vi "fit aois.vi"(5 "End frame":u32, 6 "White level":dbl format="%.2f", 7 "Header Info":T2 {"Pixel depth" items=["8 bits", "16 bits", "Float", "Complex", "RGB", "HSL"]; "time of 1st frame, \nsec since 1/1/04" format="%.2f"}, 8 "Start frame":u32, 9 "Black level":dbl format="%.2f", 10 "Acquisition refnum array":refnum<file>[](array[refnum])) -> ()   [LabVIEW 2016]
doc: "Tracks objects in successive frames of a video by calculating the parameter values that give the best fit between an analytical function and the portions of the image in selected areas of interest.\n\nOutputs an HTML report summarizing the fitting run, and a CSV-format file (which can be read by spreadsheet programs) containing the results. In addition to the parameters, each row the CSV file also contains:\n\nframe -- frame number\naoi -- aoi number\ntime -- time in milliseconds\nmse -- mean square error of the fit (or -1 if it didn't fit)\nintegral -- sum of the pixels in the aoi"
uses:
  Header file data.ctl
  Seq file v 1/Offset table.ctl
  Seq file v 1/Offset.ctl
  Seq file v 1/file number.ctl
  Parameter array.ctt
  Fit type setup.ctt
  <vilib>/Utility/NIReport.llb/HTML Report Text Alignment.ctl
  <vilib>/Utility/NIReport.llb/HTML Report Image Alignment.ctl
  AOI List Globals.vi
  GLIMPSE Globals.vi
  <vilib>/Utility/NIReport.llb/Append Report Text (str wrap).vi
  <vilib>/Utility/NIReport.llb/Append Image to Report (string wrap).vi
  <vilib>/Utility/NIReport.llb/NI_report.lvclass
  <vilib>/vision/NI_Vision_Development_Module.lvlib
  <vilib>/Utility/NIReport.llb/NI_ReportGenerationCore.lvlib
panel:
  in  "Write record when no fit?":bool=TRUE
  out "Fit":dbl[](array[numeric])
  in  "max iterations":i32=200
  in  "Update graphics?":bool=TRUE
  in  "Fit type":u16(ring) items=["2D Gaussian", "AOI Stats Only", "2D Gaussian 2 width", "Difference of Offset Gaussians (DIC)"]
  in  "Move AOIs?":bool=TRUE
  out "Last error":string
  in  "Parameters":T1=[{"Name"="bk", "Specify IV?"=TRUE, "Initial Val."=-30000.0, "Lower lim."=-32768.0, "Upper lim."=32767.0, "Fit?"=TRUE}, {"Name"="ht", "Specify IV?"=TRUE, "Initial Val."=1000.0, "Lower lim."=1.0, "Upper lim."=65000.0, "Fit?"=TRUE}, {"Name"="xc", "Specify IV?"=TRUE, "Initial Val."=10.0, "Lower lim."=0.0, "Upper lim."=512.0, "Fit?"=TRUE}, {"Name"="yc", "Specify IV?"=TRUE, "Initial Val."=10.0, "Lower lim."=0.0, "Upper lim."=512.0, "Fit?"=TRUE}, {"Name"="wi", "Specify IV?"=TRUE, "Initial Val."=2.0, "Lower lim."=0.5, "Upper lim."=20.0, "Fit?"=TRUE}] {"Upper lim." format="%.2f"; "Lower lim." format="%.2f"; "Initial Val." format="%.2f"}
  out "MSEs":dbl[](graph)
  in  "Go":bool
  out "AOI Number":i32(slide) scale=1.0..2.0
  out "Frame Number":i32(slide) scale=1.0..4390.0
  in  "stop":bool
  # "These parameters not for interactive use"
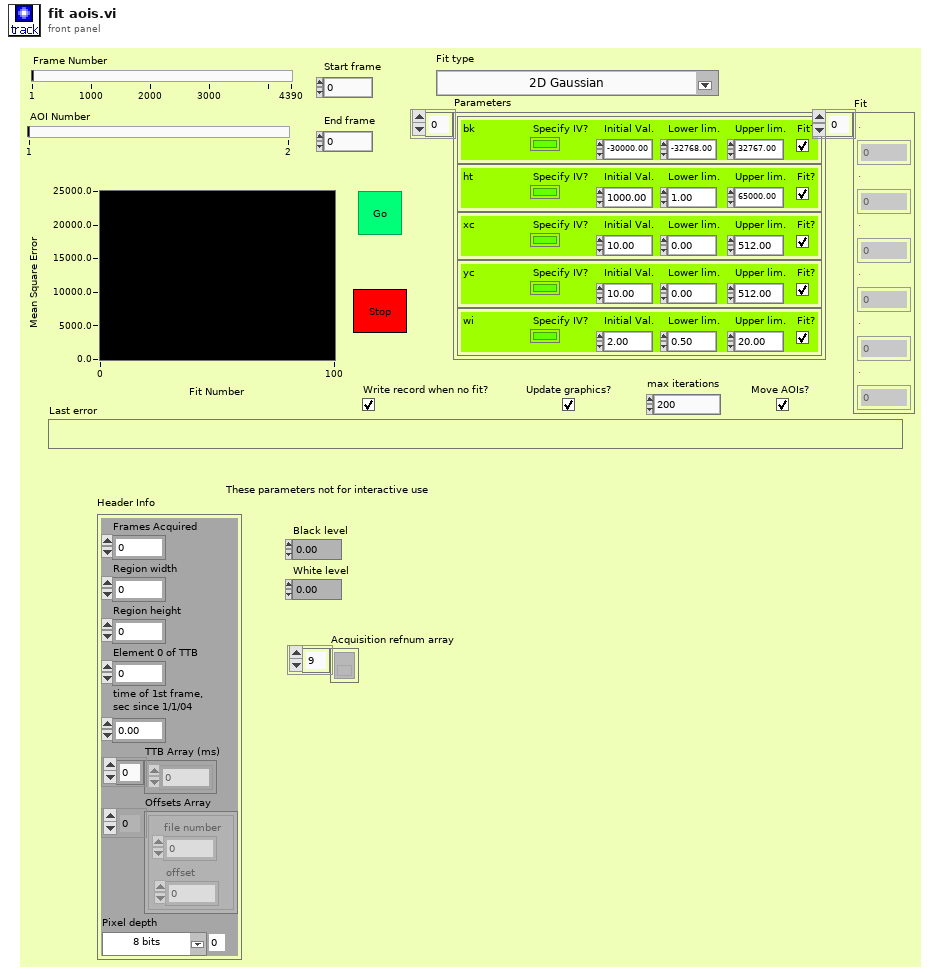
[diagram p1: front panel]
types:
  T1 = typedef "Parameter array.ctt" = cluster{"Name":string, "Specify IV?":bool, "Initial Val.":dbl, "Lower lim.":dbl, "Upper lim.":dbl, "Fit?":bool}[]
  T2 = typedef "Header file data.ctl" = cluster{"Frames Acquired":u32, "Region width":i32, "Region height":i32, "Element 0 of TTB":u32, "time of 1st frame, \nsec since 1/1/04":dbl, "TTB Array (ms)":u32[], "Offsets Array":T3, "Pixel depth":u32}
  T3 = typedef "Offset table.ctl" = cluster{"offset":T4, "file number":T5}[]
  T4 = typedef "Offset.ctl" = i32
  T5 = typedef "file number.ctl" = u8
  T6 = cluster{"Name":string, "Initial val.":dbl, "Fit?":bool}[][]
  T7 = typedef "Fit type setup.ctt" = cluster{"Fit type":string, "derivative":u16, "Parameters":T1}
  T8 = enum16{"open", "open or create", "create or replace", "create", "open (read only)"}
  T9 = typedef "IMAQ Image.ctl" = refnum<image>
  T10 = typedef "Generate Report Object Reference.ctl" = refnum<class "NI_report.lvclass">
  T11 = typedef "NI_ReportGenerationCore.lvlib/HTML Report Image Alignment.ctl" = enum16{"(default)", "LEFT", "RIGHT", "TOP", "TEXTTOP", "MIDDLE", "ABSMIDDLE", "BASELINE", "BOTTOM", "ABSBOTTOM"}
  T12 = typedef "NI_ReportGenerationCore.lvlib/HTML Report Text Alignment.ctl" = enum16{"(default)", "LEFT", "CENTER", "RIGHT"}
  T13 = cluster{"Name":string, "Initial val.":dbl, "Fit?":bool}[]
  T14 = cluster{"Name":string, "Initial Val.":dbl, "Fit?":bool}
  T15 = cluster{"Name":string, "Value":dbl, "Fit?":bool}[]
  T16 = cluster{"Name":string, "Initial Val.":dbl, "Fit?":bool}[]
  T17 = cluster{"AOI List[0]":u16, "AOI List[1]":u16, "AOI List[2]":u16, "AOI List[3]":u16, "AOI List[4]":u16, "AOI List[5]":u16, "AOI List[6]":u16, "AOI List[7]":u16, "AOI List[8]":u16}
  T18 = cluster{"AOI List[0]":u16, "AOI List[1]":u16, "AOI List[2]":u16, "AOI List[3]":u16}
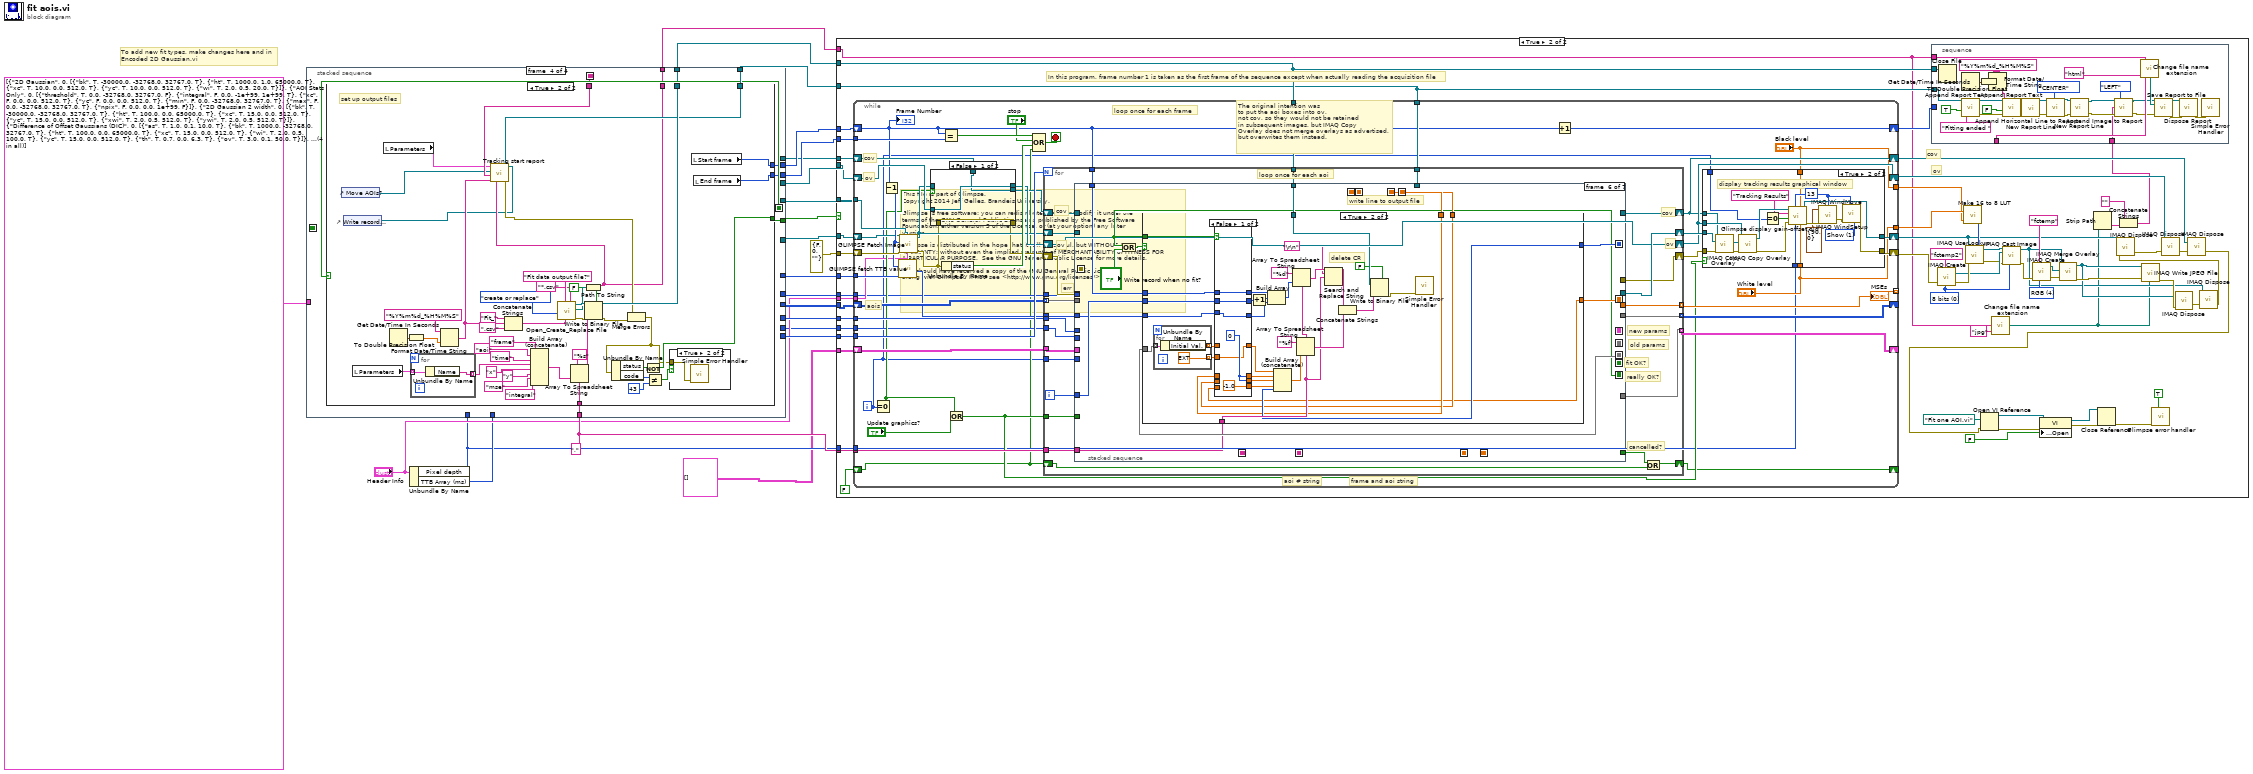
[diagram p0: block diagram]
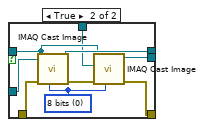
[diagram p4: hidden frame]
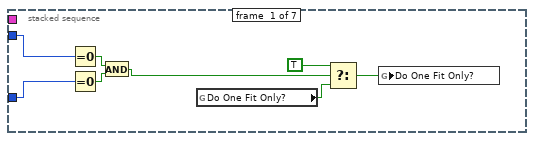
[diagram p5: hidden frame]
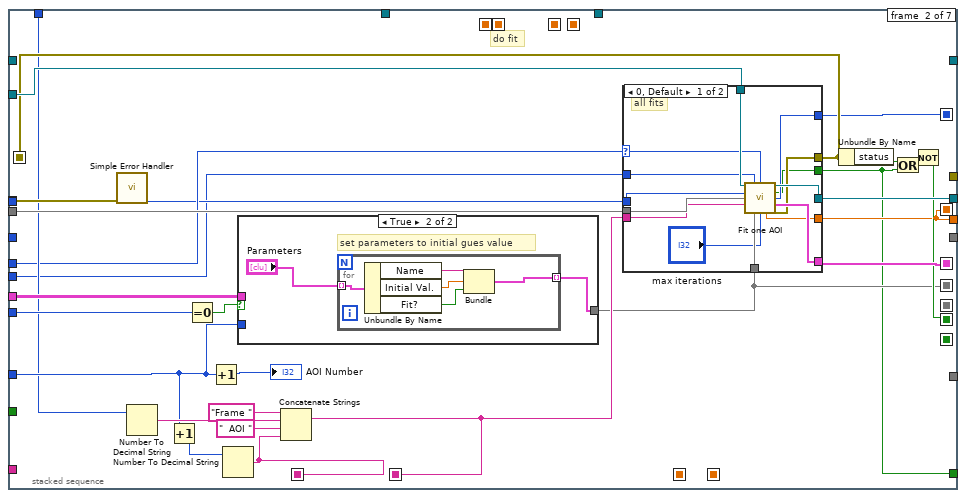
[diagram p6: hidden frame]
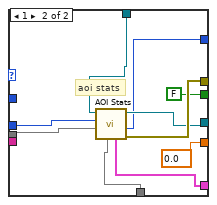
[diagram p7: hidden frame]
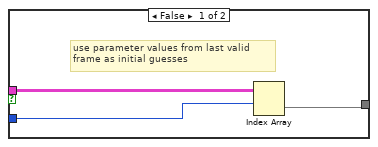
[diagram p8: hidden frame]
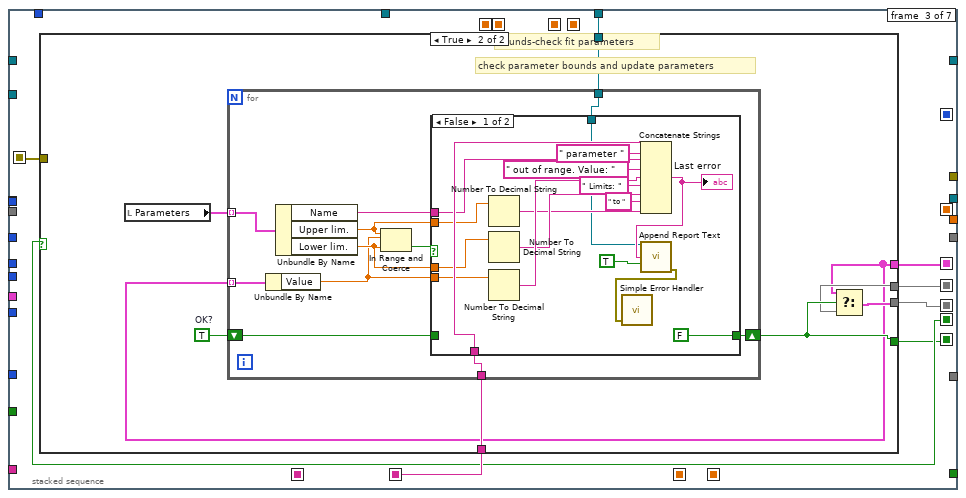
[diagram p9: hidden frame]
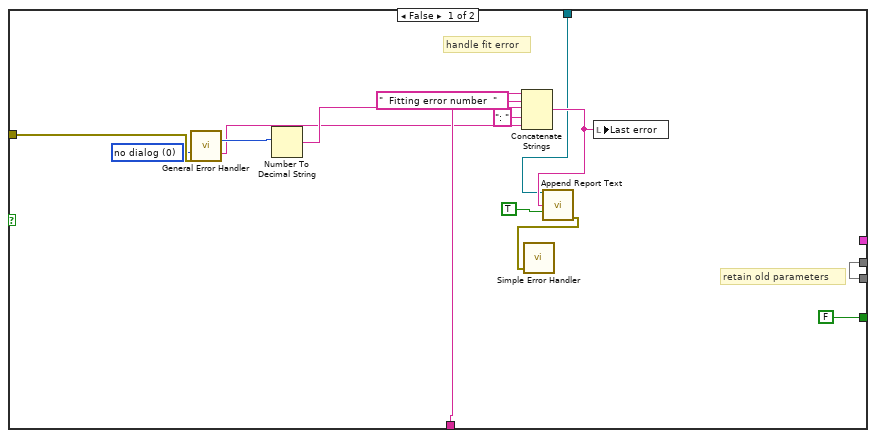
[diagram p10: hidden frame]
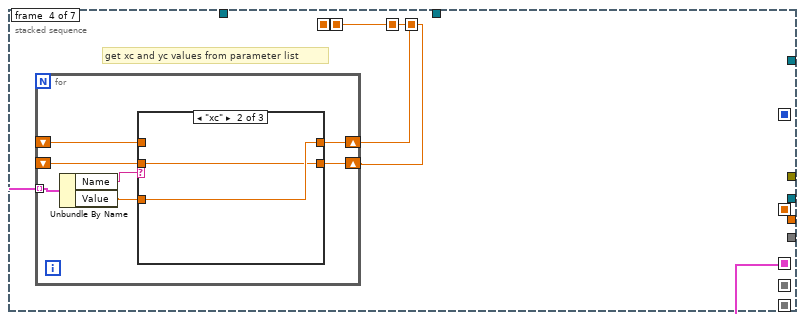
[diagram p12: hidden frame]
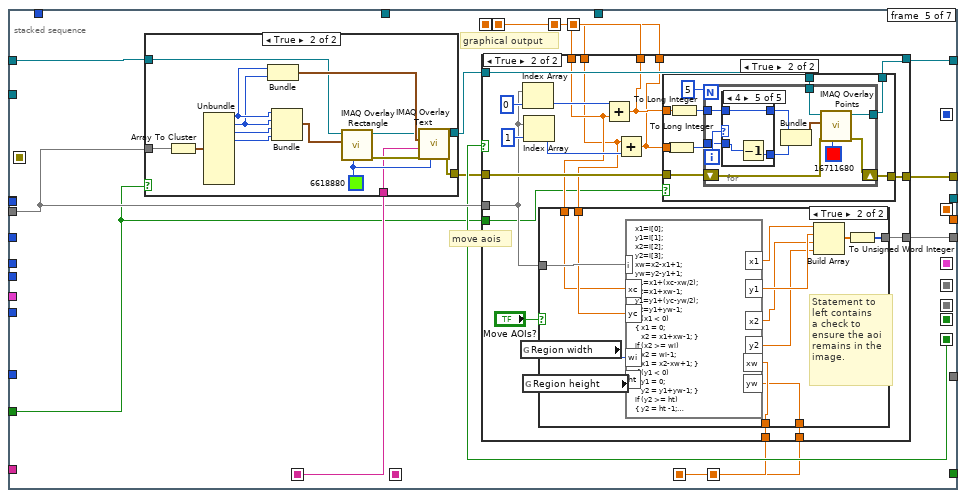
[diagram p15: hidden frame]
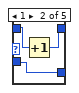
[diagram p20: hidden frame]
diagram:
  w9 = "," ("delimiter (Tab)")
  # "This file is part of Glimpse. \nCopyright 2014 Jeff Gelles, Brandeis University.    \n\nGlimpse is free software: you can redistribute it and/or modify it under the \nterms of the GNU General Public License as published by the Free Software \nFoundation, either version 3 of the License, or (at your option) any later \nversion.\n\nGlimpse is distributed in the hope that it will be useful, but WITHOUT ANY \nWARRANTY; without even the implied warranty of MERCHANTABILITY or FITNESS FOR \nA PARTICULAR PURPOSE.  See the GNU General Public License for more details.\n\nYou should have received a copy of the GNU General Public License\nalong with Glimpse.  If not, see <http://www.gnu.org/licenses/>."
  # "To add new fit types, make changes here and in\nEncoded 2D Gaussian.vi"
  n1 = Unbundle By Name("Header Info") -> ("Pixel depth"=w3:u32, "TTB Array (ms)"=w5:u32[])
  n2 = stacked-sequence {
    seq-local: [_ w43 _ _] -> [_ _ w60 _]
    seq-local: [_ _ w59 _] -> [_ _ _ w83]
    seq-local: [_ _ w55 _] -> [_ _ _ w78]
    tunnel: [_ _ _ w76] -> w23
    tunnel: [_ "Acquisition refnum array" _ _] -> w22
    tunnel: [_ w50 _ _] -> w21
    tunnel: [_ w32 _ _] -> w20
    tunnel: [_ _ _ w77] -> w19
    tunnel: [_ w47 _ _] -> w18
    tunnel: [_ _ _ w82] -> w17
    tunnel: [_ w40 _ _] -> w16
    tunnel: [_ w36 _ _] -> w14
    tunnel: [_ w33 _ _] -> w13
    tunnel: [_ _ _ w84] -> w12
    tunnel: [_ _ _ w81] -> w11
    tunnel: [_ _ _ w80] -> w10
    tunnel: w9 -> [_ _ _ w79]
    tunnel: T7[] [{"Fit type"="2D Gaussian", "derivative"=0, "Parameters"=[{"Name"="bk", "Specify IV?"=TRUE, "Initial Val."=-30000.0, "Lower lim."=-32768.0, "Upper lim."=32767.0, "Fit?"=TRUE}, {"Name"="ht", "Specify IV?"=TRUE, "Initial Val."=1000.0, "Lower lim."=1.0, "Upper lim."=65000.0, "Fit?"=TRUE}, {"Name"="xc", "Specify IV?"=TRUE, "Initial Val."=10.0, "Lower lim."=0.0, "Upper lim."=512.0, "Fit?"=TRUE}, {"Name"="yc", "Specify IV?"=TRUE, "Initial Val."=10.0, "Lower lim."=0.0, "Upper lim."=512.0, "Fit?"=TRUE}, {"Name"="wi", "Specify IV?"=TRUE, "Initial Val."=2.0, "Lower lim."=0.5, "Upper lim."=20.0, "Fit?"=TRUE}]}, {"Fit type"="AOI Stats Only", "derivative"=0, "Parameters"=[{"Name"="threshold", "Specify IV?"=TRUE, "Initial Val."=0.0, "Lower lim."=-32768.0, "Upper lim."=32767.0, "Fit?"=FALSE}, {"Name"="integral", "Specify IV?"=FALSE, "Initial Val."=0.0, "Lower lim."=-1e+99, "Upper lim."=1e+99, "Fit?"=TRUE}, {"Name"="xc", "Specify IV?"=FALSE, "Initial Val."=0.0, "Lower lim."=0.0, "Upper lim."=512.0, "Fit?"=TRUE}, {"Name"="yc", "Specify IV?"=FALSE, "Initial Val."=0.0, "Lower lim."=0.0, "Upper lim."=512.0, "Fit?"=TRUE}, {"Name"="min", "Specify IV?"=FALSE, "Initial Val."=0.0, "Lower lim."=-32768.0, "Upper lim."=32767.0, "Fit?"=TRUE}, {"Name"="max", "Specify IV?"=FALSE, "Initial Val."=0.0, "Lower lim."=-32768.0, "Upper lim."=32767.0, "Fit?"=TRUE}, {"Name"="npix", "Specify IV?"=FALSE, "Initial Val."=0.0, "Lower lim."=0.0, "Upper lim."=1e+99, "Fit?"=FALSE}]}, {"Fit type"="2D Gaussian 2 width", "derivative"=0, "Parameters"=[{"Name"="bk", "Specify IV?"=TRUE, "Initial Val."=-30000.0, "Lower lim."=-32768.0, "Upper lim."=32767.0, "Fit?"=TRUE}, {"Name"="ht", "Specify IV?"=TRUE, "Initial Val."=100.0, "Lower lim."=0.0, "Upper lim."=65000.0, "Fit?"=TRUE}, {"Name"="xc", "Specify IV?"=TRUE, "Initial Val."=15.0, "Lower lim."=0.0, "Upper lim."=512.0, "Fit?"=TRUE}, {"Name"="yc", "Specify IV?"=TRUE, "Initial Val."=15.0, "Lower lim."=0.0, "Upper lim."=512.0, "Fit?"=TRUE}, {"Name"="xwi", "Specify IV?"=TRUE, "Initial Val."=2.0, "Lower lim."=0.5, "Upper lim."=512.0, "Fit?"=TRUE}, {"Name"="ywi", "Specify IV?"=TRUE, "Initial Val."=2.0, "Lower lim."=0.5, "Upper lim."=512.0, "Fit?"=TRUE}]}, {"Fit type"="Difference of Offset Gaussians (DIC)", "derivative"=0, "Parameters"=[{"Name"="as", "Specify IV?"=TRUE, "Initial Val."=1.0, "Lower lim."=0.1, "Upper lim."=10.0, "Fit?"=TRUE}, {"Name"="bk", "Specify IV?"=TRUE, "Initial Val."=1000.0, "Lower lim."=-32768.0, "Upper lim."=32767.0, "Fit?"=TRUE}, {"Name"="ht", "Specify IV?"=TRUE, "Initial Val."=100.0, "Lower lim."=0.0, "Upper lim."=65000.0, "Fit?"=TRUE}, {"Name"="xc", "Specify IV?"=TRUE, "Initial Val."=15.0, "Lower lim."=0.0, "Upper lim."=512.0, "Fit?"=TRUE}, {"Name"="wi", "Specify IV?"=TRUE, "Initial Val."=2.0, "Lower lim."=0.5, "Upper lim."=100.0, "Fit?"=TRUE}, {"Name"="yc", "Specify IV?"=TRUE, "Initial Val."=15.0, "Lower lim."=0.0, "Upper lim."=512.0, "Fit?"=TRUE}, {"Name"="th", "Specify IV?"=TRUE, "Initial Val."=0.7, "Lower lim."=0.0, "Upper lim."=6.3, "Fit?"=TRUE}, {"Name"="ov", "Specify IV?"=TRUE, "Initial Val."=3.0, "Lower lim."=0.1, "Upper lim."=50.0, "Fit?"=TRUE}]}] -> [w25 _ w57 _]
    tunnel: [_ _ w56 _] -> w7
    tunnel: w3 -> [_ w31 _ _]
    tunnel: w5 -> [_ w32 _ _]
    tunnel: [_ w31 _ _] -> w4
    tunnel: [_ _ w53 _] -> w1
    frame #0 {
      n3 = for {
        tunnel: w25 -> [w29] mode=indexing
        tunnel: [w28] -> w24 mode=indexing
        n4 = Unbundle By Name(w29) -> ("Fit type"=w28:string)
      }
      n5 = property on="Fit type" class="Ring (strict)"("Strings []"=w24) -> ()  [unwired: 2 in, 2 out]
      n6 = local write "stop"(FALSE ("stop")) -> ()
      n7 = local write "Go"(FALSE ("stop")) -> ()
    }
    frame #1 {
      w34 = u32 0 items=["8 bits", "16 bits", "Float", "Complex", "RGB", "HSL"] ("Image Type")
      n8 = global read "AOI List Globals.vi" "AOI List"() -> (w47:u16[][])
      n9 = property on="Frame Number" class="Slide (strict)"("Scale.Range:Minimum"="Start frame", "Scale.Range:Maximum"="End frame") -> ()  [unwired: 2 in, 2 out]
      n10 = call "Position calling vi to LR 2.vi"("Corner"=enum16{"LR", "LL"}."LL") -> ()  [unwired: 1 in, 4 out]
      n11 = call "IMAQ Create"("Image Name"="cum overlay", "Image Type"=w34) -> ("New Image"=w33:T9)  [unwired: 2 in, 2 out]
      n12 = Array Size(array=w47) -> (size(s)=w46:i32[])
      n13 = Index Array(array=w46, index=0) -> (element=w40:i32)
      n14 = local write "Frame Number"(0 ("Frame Number")) -> ()
      n15 = local write "AOI Number"(0 ("AOI Number")) -> ()
      n16 = call "IMAQ Create"("Image Name"="overlay", "Image Type"=w34) -> ("New Image"=w36:T9, "error out"=w37:errorcluster)  [unwired: 2 in, 1 out]
      n17 = property on="AOI Number" class="Slide (strict)"("Scale.Range:Maximum"=w40, "Scale.Range:Minimum"=1.0) -> ()  [unwired: 2 in, 2 out]
      n18 = call "IMAQ Create"("Image Name"="fitimage", "Image Type"=w31, "error in (no error)"=w37) -> ("New Image"=w50:T9, "error out"=w44:errorcluster)  [unwired: 1 in, 1 out]
      n19 = Unbundle By Name(w44) -> ("status"=w43:bool)
      n20 = call <vilib>:"Simple Error Handler.vi"("error in (no error)"=w44) -> ()  [unwired: 1 in, 8 out]
    }
    frame #2 {
      n21 = local read "Fit type"() -> (w54:u16)
      n22 = while {
        tunnel: w60 -> [w70]
        tunnel: ["Go"] -> w59
        shift-right: [w61] -> w56
        shift-left: w54 -> [w65]
        tunnel: w57 -> [w62]
        stop <- w69 stop-if-true
        n23 = To Word Integer(number="Fit type") -> (16bit integer=w61:i16)
        n24 = local read "stop"() -> (w71:bool)
        n25 = Not Equal?(x=w61, y=w65) -> (x != y?=w63:bool)
        n26 = Or(x=w71, y=w70) -> (x .or. y?=w67:bool)
        n27 = Or(x="Go", y=w67) -> (x .or. y?=w69:bool)
        n28 = case shown="True" w63 {
          tunnel: w62 -> [_ w75]
          tunnel: w61 -> [_ w74]
          frame False {
          }
          frame True {
            n29 = Index Array(array=w75, index=w74) -> (element=w73:T7)
            n30 = Unbundle By Name(w73) -> ("Parameters"=w72:T1)
            n31 = local write "Parameters"(w72) -> ()
          }
        }
        n32 = Wait (ms)(milliseconds to wait=u32 300) -> ()  [unwired: 1 out]
      }
      n33 = Index Array(array=w57, index=w56) -> (element=w58:T7)
      n34 = Unbundle By Name(w58) -> ("Fit type"=w55:string, "derivative"=w53:u16)
    }
    frame #3 {
      n35 = case shown="True" w83 {
        selector: w83 -> [w85 _]
        tunnel: [_ w97] -> w84
        tunnel: [w85 w117] -> w82
        tunnel: [_ w104] -> w81
        tunnel: [_ w92] -> w80
        tunnel: w79 -> [_ w102]
        tunnel: w78 -> [_ w95]
        tunnel: [_ w89] -> w77
        tunnel: [_ w88] -> w76
        frame False {
        }
        frame True {
          # "set up output files"
          n36 = control-ref of="Move AOIs?"() -> (w94:refnum<vi>)
          n37 = control-ref of="Write record when no fit?"() -> (w87:refnum<vi>)
          n38 = local read "Parameters"() -> (w116:T1)
          n39 = local read "Parameters"() -> (w93:T1)
          n40 = Get Date/Time In Seconds() -> (seconds since 1Jan1904=w91:timestamp)
          n41 = To Double Precision Float(number=w91) -> (double precision float=w129:dbl)
          n42 = for {
            tunnel: w116 -> [w131] mode=indexing
            tunnel: [w130] -> w110 mode=indexing
            n43 = Unbundle By Name(w131) -> ("Name"=w130:string)
          }
          n44 = Format Date/Time String(time format string (%c)="%Y%m%d_%H%M%S", seconds (now)=w129) -> (date/time string=w124:string)  [unwired: 1 out]
          n45 = Concatenate Strings("Fit_", w124, ".csv" ("string")) -> (w122:string)
          n46 = Build Array (concatenate)("frame", "aoi", "time", w110, "x", "y", "mse", "integral" ("element")) -> (w112:string[])
          n47 = call <vilib>:"Open_Create_Replace File.vi"("pattern"="*.csv", "default name"=w122, "prompt"="Fit data output file?", "function (open:0)"=T8."create or replace") -> ("error out"=w103:errorcluster, "new file path"=w107:path, "refnum"=w114:refnum<file>)  [unwired: 3 in, 2 out]
          n48 = Array To Spreadsheet String(delimiter (Tab)=w102, array=w112, 3:"%s" ("format string")) -> (spreadsheet string=w113:string)
          n49 = Path To String(path=w107) -> (string=w92:string)
          n50 = call "Tracking start report.vi"("Write record when no fit?"=w87, "Filename"=w92, "date/time string"=w124, "Fit type"=w95, "Move AOIs?"=w94, "Parameters"=w93) -> ("error out (no error)"=w98:errorcluster, "report out"=w97:T10)  [unwired: 1 out]
          n51 = Write to Binary File(file (use dialog)=w114, data=w113, error in=w103, 5:FALSE ("prepend array or string size? (T)")) -> (refnum out=w104:refnum<file>, error out=w105:errorcluster)  [unwired: 3 out]
          n52 = Merge Errors(w98, w105) -> (w106:errorcluster)
          n53 = Unbundle By Name(w106) -> ("status"=w118:bool, "code"=w121:i32)
          n54 = Not(x=w118) -> (.not. x?=w117:bool)
          n55 = Not Equal?(x=w121, y=43) -> (x != y?=w119:bool)
          n56 = case shown="True" w119 {
            tunnel: w106 -> [_ w132]
            frame False {
            }
            frame True {
              n57 = call <vilib>:"Simple Error Handler.vi"("error in (no error)"=w132) -> ()  [unwired: 1 in, 8 out]
            }
          }
          n58 = local read "Start frame"() -> (w88:u32)
          n59 = local read "End frame"() -> (w89:u32)
        }
      }
    }
  }
  n60 = case shown="True" w17 {
    tunnel: w23 -> [_ w194]
    tunnel: w22 -> [_ w193]
    tunnel: w21 -> [_ w184]
    tunnel: w20 -> [_ w192]
    tunnel: w19 -> [_ w191]
    tunnel: w18 -> [_ w179]
    tunnel: T6 [] ("Array") -> [_ w190]
    tunnel: w16 -> [_ w189]
    tunnel: errorcluster {"status"=FALSE, "code"=0, "source"=""} ("error out") -> [_ w188]
    tunnel: w14 -> [_ w186]
    tunnel: w13 -> [_ w182]
    tunnel: w12 -> [_ w176]
    tunnel: w11 -> [_ w177]
    tunnel: w10 -> [_ w151]
    tunnel: w9 -> [_ w175]
    tunnel: w7 -> [_ w149]
    tunnel: "Header Info" -> [_ w140]
    tunnel: w4 -> [_ w139]
    tunnel: w3 -> [_ w138]
    tunnel: w1 -> [_ w137]
    frame False {
    }
    frame True {
      w162 = u32 0 items=["8 bits", "16 bits", "Float", "Complex", "RGB", "HSL"] ("Image Type")
      w174 = u32 4 items=["8 bits", "16 bits", "Float", "Complex", "RGB", "HSL"] ("Image Type")
      # "cov"
      # "ov"
      # "In this program, frame number 1 is taken as the first frame of the sequence except when actually reading the acquisition file"
      n61 = while {
        tunnel: [w261] -> _ mode=indexing
        shift-right: [w272] -> w178
        shift-left: w194 -> [w240]
        tunnel: w193 -> [w268]
        tunnel: w192 -> [w267]
        tunnel: w191 -> [w266]
        shift-right: [w265] -> _
        shift-left: w190 -> [w264]
        shift-right: [w236] -> w167
        shift-left: w188 -> [w263]
        tunnel: w189 -> [w259]
        shift-right: [w248] -> w185
        shift-left: w186 -> [w256]
        shift-right: [w235] -> w165
        shift-left: w184 -> [w257]
        shift-right: [w247] -> w180
        shift-left: w182 -> [w250]
        shift-right: [w244] -> _
        shift-left: w179 -> [w246]
        tunnel: w176 -> [w245]
        tunnel: w177 -> [w242]
        tunnel: w175 -> [w241]
        tunnel: ["White level"] -> w169
        tunnel: ["Black level"] -> w168
        tunnel: w149 -> [w239]
        tunnel: w140 -> [w231]
        tunnel: w139 -> [w230]
        tunnel: w138 -> [w229]
        tunnel: w137 -> [w228]
        shift-right: [w227] -> _
        shift-left: FALSE -> [w226]
        i -> [w225]
        stop <- w269 stop-if-true
        # "frame and aoi string"
        # "aois"
        # "aoi # string"
        # "The original intention was \nto put the aoi boxes into ov,\nnot cov, so they would not be retained \nin subsequent images, but IMAQ Copy \nOverlay does not merge overlays as advertised,\nbut overwrites them instead."
        # "cov"
        # "ov"
        # "loop once for each frame"
        n62 = Equal To 0?(x=w225) -> (x = 0?=w237:bool)
        n63 = Decrement(x=w240) -> (x-1=w260:u32)
        n64 = call "GLIMPSE fetch TTB value.vi"("Array of TTB Values (ms)"=w267, "Logical Frame Number\n(starting with zero)"=w260) -> ("TTB value out"=w243:u32)  [unwired: 6 out]
        n65 = call "GLIMPSE Fetch Image.vi"("Header file data"=w231, "Acqisition files refnums"=w268, "error in"=w263, "Logical Frame Number\n(starting with zero)"=w260, "Image In"=w257) -> ("error out"=w253:errorcluster, "Image Out"=w254:T9)  [unwired: 4 in, 1 out]
        n66 = case shown="False" w237 {
          tunnel: w256 -> [w297 w307]
          tunnel: [w297 w306] -> w255
          tunnel: w254 -> [_ w302]
          tunnel: w253 -> [w298 w305]
          tunnel: [w298 w303] -> w252
          tunnel: w250 -> [w296 w301]
          tunnel: [w296 w300] -> w249
          frame False {
          }
          frame True {
            w299 = u32 0 items=["8 bits", "16 bits", "Float", "Complex", "RGB", "HSL"] ("Image Type")
            n67 = call "IMAQ Cast Image"("Image Type"=w299, "error in (no error)"=w305, "Image Dst"=w307, "Image Src"=w302) -> ("error out"=w304:errorcluster, "Image Dst Out"=w306:T9)  [unwired: 2 in, 4 out]
            n68 = call "IMAQ Cast Image"("Image Type"=w299, "error in (no error)"=w304, "Image Dst"=w301, "Image Src"=w302) -> ("error out"=w303:errorcluster, "Image Dst Out"=w300:T9)  [unwired: 2 in, 4 out]
          }
        }
        n69 = Equal?(x=w240, y=w266) -> (x = y?=w271:bool)
        n70 = Unbundle By Name(w253) -> ("status"=w262:bool)
        n71 = Or(x=w237, y="Update graphics?") -> (x .or. y?=w234:bool)
        n72 = Compound Arithmetic op=OR(w271, "stop", w262, w226) -> (w269:bool)
        n73 = for {
          N: w259 -> [_]
          tunnel: [w320] -> w265 mode=indexing
          tunnel: [w333] -> w261 mode=indexing
          tunnel: w246 -> [w329] mode=indexing
          tunnel: w264 -> [w332]
          tunnel: w225 -> [w330]
          shift-right: [w324] -> w258
          shift-left: w252 -> [w327]
          shift-right: [w326] -> w251
          shift-left: w254 -> [w328]
          shift-right: [w323] -> w248
          shift-left: w255 -> [w323]
          shift-right: [w325] -> w247
          shift-left: w249 -> [w322]
          tunnel: w245 -> [w321]
          tunnel: [w319] -> w244 mode=indexing
          tunnel: w243 -> [w318]
          tunnel: w242 -> [w317]
          tunnel: w241 -> [w316]
          tunnel: w240 -> [w315]
          tunnel: w239 -> [w314]
          tunnel: w234 -> [w313]
          tunnel: w230 -> [w312]
          tunnel: w228 -> [w311]
          shift-right: [w310] -> w227
          shift-left: w226 -> [w308]
          i -> [w331]
          # "cancelled?"
          # "really OK?"
          # "old params"
          # "new params"
          # "fit OK?"
          # "err"
          # "cov"
          # "cov"
          # "ov"
          # "ov"
          # "loop once for each aoi"
          n74 = stacked-sequence {
            seq-local: [_ w358 _ _ _ _ _] -> [_ _ _ _ w493 _ _]
            seq-local: [_ w357 _ _ _ _ _] -> [_ _ w411 w465 _ _ _]
            seq-local: [_ w351 _ _ _ _ _] -> [_ _ w408 _ _ _ _]
            seq-local: [_ w355 _ _ _ _ _] -> [_ _ w406 _ _ _ _]
            seq-local: [_ w354 _ _ _ _ _] -> [_ _ w410 _ _ _ _]
            seq-local: [_ w353 _ _ _ _ _] -> [_ _ w407 _ _ _ _]
            seq-local: [_ _ w405 _ _ _ _] -> [_ _ _ _ w488 w582 w650]
            seq-local: [_ _ w404 _ _ _ _] -> [_ _ _ _ _ w592 w644]
            seq-local: [_ w350 _ _ _ _ _] -> [_ _ _ _ _ w591 _]
            seq-local: [_ _ _ _ w485 _ _] -> [_ _ _ _ _ w588 _]
            seq-local: [_ _ _ _ w484 _ _] -> [_ _ _ _ _ w587 _]
            seq-local: [_ _ _ w464 _ _ _] -> [_ _ _ _ w483 _ _]
            seq-local: [_ _ _ w463 _ _ _] -> [_ _ _ _ w482 _ _]
            seq-local: [_ _ _ _ w481 _ _] -> [_ _ _ _ _ _ w646]
            seq-local: [_ _ _ _ w480 _ _] -> [_ _ _ _ _ _ w645]
            seq-local: [_ w345 _ _ _ _ _] -> [_ _ _ _ _ w585 _]
            tunnel: [_ w350 _ _ _ _ _] -> w333
            tunnel: w332 -> [_ w368 _ _ _ _ _]
            tunnel: w331 -> [w334 w363 _ _ _ w594 _]
            tunnel: w330 -> [w335 w362 _ _ _ _ _]
            tunnel: w329 -> [_ w359 _ _ w491 _ _]
            tunnel: w328 -> [_ w356 _ _ _ _ _]
            tunnel: w327 -> [_ w352 _ _ _ _ _]
            tunnel: [_ w360 _ _ _ _ _] -> w326
            tunnel: [_ _ _ _ w489 _ _] -> w325
            tunnel: [_ _ _ _ w490 _ _] -> w324
            tunnel: w322 -> [_ _ _ _ w492 _ _]
            tunnel: w321 -> [_ _ w409 _ _ _ _]
            tunnel: [_ _ _ _ _ _ w647] -> w320
            tunnel: [_ _ _ _ w486 _ _] -> w319
            tunnel: w318 -> [_ _ _ _ _ w593 _]
            tunnel: w317 -> [_ _ _ _ _ w590 _]
            tunnel: w316 -> [_ _ _ _ _ w589 _]
            tunnel: w315 -> [_ w349 _ _ _ w586 _]
            tunnel: w314 -> [_ w348 _ _ _ _ _]
            tunnel: w313 -> [_ _ _ _ w479 _ _]
            tunnel: w312 -> [_ w347 _ _ _ _ _]
            tunnel: w311 -> [_ w346 _ _ _ _ _]
            tunnel: [_ w342 _ _ _ _ _] -> w309
            frame #0 {
              n75 = Equal To 0?(x=w335) -> (x = 0?=w336:bool)
              n76 = Equal To 0?(x=w334) -> (x = 0?=w341:bool)
              n77 = And(x=w336, y=w341) -> (x .and. y?=w340:bool)
              n78 = global read "GLIMPSE Globals.vi" "Do One Fit Only?"() -> (w338:bool)
              n79 = Select(t=TRUE, s=w340, f=w338) -> (s? t:f=w339:bool)
              n80 = global write "GLIMPSE Globals.vi" "Do One Fit Only?"(w339) -> ()
            }
            frame #1 {
              # "do fit"
              n81 = call <vilib>:"Simple Error Handler.vi"("error in (no error)"=w352) -> ()  [unwired: 1 in, 8 out]
              n82 = Number To Decimal String(number=w349) -> (decimal integer string=w365:string)  [unwired: 1 out]
              n83 = Increment(x=w363) -> (x+1=w361:i32)
              n84 = Equal To 0?(x=w362) -> (x = 0?=w367:bool)
              n85 = Increment(x=w363) -> (x+1=→"AOI Number":i32)
              n86 = Number To Decimal String(number=w361) -> (decimal integer string=w358:string)  [unwired: 1 out]
              n87 = case shown="True" w367 {
                tunnel: [w394 w397] -> w353
                tunnel: w368 -> [w396 _]
                tunnel: w363 -> [w395 _]
                frame False {
                  # "use parameter values from last valid\nframe as initial guesses"
                  n88 = Index Array(array=w396, index (row)=w395) -> (element=w394:T13)  [unwired: 1 in]
                }
                frame True {
                  # "set parameters to initial gues value"
                  n89 = for {
                    tunnel: "Parameters" -> [w403] mode=indexing
                    tunnel: [w401] -> w397 mode=indexing
                    n90 = Unbundle By Name(w403) -> ("Name"=w402:string, "Initial Val."=w400:dbl, "Fit?"=w399:bool)
                    n91 = Bundle("Name"=w402, "Initial Val."=w400, "Fit?"=w399) -> (w401:T14)  [unwired: 1 out]
                  }
                }
              }
              n92 = Concatenate Strings("Frame " ("string"), w365, "  AOI " ("string"), w358) -> (w354:string)
              n93 = case shown="0, Default" w348 {
                selector: w348 -> [w373 _]
                tunnel: w347 -> [w383 w390]
                tunnel: [w382 w387] -> w360
                tunnel: w359 -> [w381 w389]
                tunnel: [w380 w388] -> w357
                tunnel: w356 -> [w379 w391]
                tunnel: w354 -> [w378 _]
                tunnel: w353 -> [w377 w386]
                tunnel: [w376 w392] -> w351
                tunnel: [w375 0.0 ("mse")] -> w350
                tunnel: w346 -> [w372 _]
                tunnel: [w371 w385] -> w345
                tunnel: [w370 FALSE ("Cancelled?")] -> w342
                frame 0, Default {
                  # "all fits"
                  n94 = call "Fit one AOI.vi"("Image In"=w379, "derivative"=w372, "fit type"=w373, "Image Type"=w383, "AOI (l, t, r, b)"=w381, "Data ID"=w378, "Guessed"=w377, "max iterations"="max iterations") -> ("Image Out"=w382:T9, "Cancelled?"=w370:bool, "integral"=w371:i32, "Fit"=w380:T15, "mse"=w375:dbl, "error out"=w376:errorcluster)  [unwired: 1 in, 1 out]
                }
                frame 1 {
                  # "aoi stats"
                  n95 = call "AOI Stats.vi"("Params In"=w386, "AOI (l, t, r, b)"=w389, "Image Type"=w390, "Image In"=w391) -> ("error out"=w392:errorcluster, "integral"=w385:i32, "Image Out"=w387:T9, "Params out"=w388:T15)  [unwired: 1 in, 3 out]
                }
              }
              n96 = Unbundle By Name(w351) -> ("status"=w343:bool)
              n97 = Or(x=w343, y=w342) -> (x .or. y?=w344:bool)
              n98 = Not(x=w344) -> (.not. x?=w355:bool)
            }
            frame #2 {
              # "bounds-check fit parameters"
              n99 = case shown="True" w406 {
                tunnel: w411 -> [_ w426]
                tunnel: w410 -> [w419 w431]
                tunnel: w409 -> [w414 w430]
                tunnel: w408 -> [w425 _]
                tunnel: w407 -> [w413 w427]
                tunnel: [w413 w429] -> w404
                tunnel: [FALSE w428] -> w405
                frame False {
                  w424 = u16 0 items=["no dialog", "OK message", "continue or stop message"] ("type of dialog (OK msg:1)")
                  # "retain old parameters"
                  # "handle fit error"
                  n100 = call <vilib>:"General Error Handler.vi"("type of dialog (OK msg:1)"=w424, "error in (no error)"=w425) -> ("code out"=w418:i32, "message"=w416:string)  [unwired: 1 in, 11 out]
                  n101 = Number To Decimal String(number=w418) -> (decimal integer string=w417:string)  [unwired: 1 out]
                  n102 = Concatenate Strings(w419, "  Fitting error number  " ("string"), w417, ": " ("string"), w416) -> (w415:string)
                  n103 = call-poly <vilib>:"Append Report Text.vi"("report in"=w414, "text"=w415, "append on new line? (F)"=TRUE) -> ("error out"=w420:errorcluster)  [unwired: 3 in, 9 out]
                  n104 = call <vilib>:"Simple Error Handler.vi"("error in (no error)"=w420) -> ()  [unwired: 1 in, 8 out]
                  n105 = local write "Last error"(w415) -> ()
                }
                frame True {
                  w432 = TRUE  # OK?
                  # "check parameter bounds and update parameters"
                  n106 = local read "Parameters"() -> (w433:T1)
                  n107 = for {
                    tunnel: w433 -> [w444] mode=indexing
                    tunnel: w426 -> [w436] mode=indexing
                    shift-right: [w441] -> w428
                    shift-left: w432 -> [w442]
                    tunnel: w431 -> [w440]
                    tunnel: w430 -> [w435]
                    n108 = Unbundle By Name(w436) -> ("Value"=w434:dbl)
                    n109 = Unbundle By Name(w444) -> ("Name"=w439:string, "Upper lim."=w438:dbl, "Lower lim."=w437:dbl)
                    n110 = In Range and Coerce(upper limit=w438, x=w434, lower limit=w437) -> (In Range?=w443:bool)  [unwired: 1 out]
                    n111 = case shown="False" w443 {
                      tunnel: w442 -> [_ w462]
                      tunnel: [FALSE ("OK?") w462] -> w441
                      tunnel: w440 -> [w459 _]
                      tunnel: w439 -> [w457 _]
                      tunnel: w438 -> [w454 _]
                      tunnel: w437 -> [w453 _]
                      tunnel: w434 -> [w452 _]
                      tunnel: w435 -> [w445 _]
                      frame False {
                        n112 = Number To Decimal String(number=w454) -> (decimal integer string=w448:string)  [unwired: 1 out]
                        n113 = Number To Decimal String(number=w453) -> (decimal integer string=w450:string)  [unwired: 1 out]
                        n114 = Number To Decimal String(number=w452) -> (decimal integer string=w451:string)  [unwired: 1 out]
                        n115 = Concatenate Strings(w459, " parameter " ("string"), w457, " out of range. Value: " ("string"), w451, " Limits: " ("string"), w450, " to " ("string"), w448) -> (w447:string)
                        "Last error" <- w447
                        n116 = call-poly <vilib>:"Append Report Text.vi"("report in"=w445, "text"=w447, "append on new line? (F)"=TRUE) -> ("error out"=w446:errorcluster)  [unwired: 3 in, 9 out]
                        n117 = call <vilib>:"Simple Error Handler.vi"("error in (no error)"=w446) -> ()  [unwired: 1 in, 8 out]
                      }
                      frame True {
                      }
                    }
                  }
                  n118 = Select(t=w426, s=w428, f=w427) -> (s? t:f=w429:T16)
                }
              }
            }
            frame #3 {
              # "get xc and yc values from parameter list"
              n119 = for {
                tunnel: w465 -> [w472] mode=indexing
                shift-right: [w469] -> w464
                shift-left: _ -> [w468]
                shift-right: [w466] -> w463
                shift-left: _ -> [w467]
                n120 = Unbundle By Name(w472) -> ("Name"=w471:string, "Value"=w470:dbl)
                n121 = case shown="\"xc\"" w471 {
                  tunnel: w470 -> [_ w476 w478]
                  tunnel: [w474 w476 w477] -> w469
                  tunnel: w468 -> [w474 _ w477]
                  tunnel: w467 -> [w473 w475 _]
                  tunnel: [w473 w475 w478] -> w466
                  frame Default {
                  }
                  frame "xc" {
                  }
                  frame "yc" {
                  }
                }
              }
            }
            frame #4 {
              # "move aois"
              # "graphical output"
              n122 = case shown="True" w479 {
                tunnel: [w495 w501] -> w494
                tunnel: w493 -> [_ w499]
                tunnel: w492 -> [w495 w498]
                tunnel: w491 -> [_ w497]
                tunnel: [_ w496] -> w487
                frame False {
                }
                frame True {
                  w502 = u32 6618880 ("Color")
                  n123 = Array To Cluster(array=w497) -> (cluster=w510:T17)
                  n124 = Unbundle(w510) -> ("AOI List[0]"=w505:u16, "AOI List[1]"=w504:u16, "AOI List[2]"=w509:u16, "AOI List[3]"=w508:u16)  [unwired: 5 out]
                  n125 = Bundle("AOI List[0]"=w505, "AOI List[1]"=w504) -> (w503:cluster{"AOI List[0]":u16, "AOI List[1]":u16})  [unwired: 1 out]
                  n126 = Bundle("AOI List[0]"=w505, "AOI List[1]"=w504, "AOI List[2]"=w509, "AOI List[3]"=w508) -> (w507:T18)  [unwired: 1 out]
                  n127 = call "IMAQ Overlay Rectangle"("Color"=w502, "Rectangle"=w507, "Image"=w498) -> ("error out"=w506:errorcluster, "Image Out"=w500:T9)  [unwired: 3 in, 4 out]
                  n128 = call "IMAQ Overlay Text"("Text Color (black)"=w502, "error in (no error)"=w506, "String"=w499, "Origin"=w503, "Image"=w500) -> ("error out"=w496:errorcluster, "Image Out"=w501:T9)  [unwired: 3 in, 2 out]
                }
              }
              n129 = case shown="True" w488 {
                tunnel: w494 -> [w513 w527]
                tunnel: w491 -> [w511 w522]
                tunnel: [w512 w526] -> w490
                tunnel: [w513 w525] -> w489
                tunnel: w487 -> [w512 w524]
                tunnel: [w511 w521] -> w486
                tunnel: [_ w520] -> w485
                tunnel: [_ w519] -> w484
                tunnel: w483 -> [_ w518]
                tunnel: w482 -> [_ w517]
                tunnel: [_ w516] -> w481
                tunnel: [_ w515] -> w480
                tunnel: w479 -> [_ w514]
                frame False {
                }
                frame True {
                  n130 = Index Array(array=w522, index=0) -> (element=w528:u16)
                  n131 = Index Array(array=w522, index=1) -> (element=w529:u16)
                  n132 = case shown="True" "Move AOIs?" {
                    tunnel: w522 -> [w568 w581]
                    tunnel: [w568 w575] -> w521
                    tunnel: w517 -> [_ w574]
                    tunnel: w518 -> [_ w573]
                    tunnel: [_ w572] -> w516
                    tunnel: [_ w571] -> w515
                    frame False {
                    }
                    frame True {
                      # "Statement to \nleft contains\na check to\nensure the aoi\nremains in the\nimage."
                      n133 = global read "GLIMPSE Globals.vi" "Region width"() -> (w570:u16)
                      n134 = global read "GLIMPSE Globals.vi" "Region height"() -> (w569:u16)
                      n135 = formula code="x1=i[0];\ny1=i[1];\nx2=i[2];\ny2=i[3];\nxw=x2-x1+1;\nyw=y2-y1+1;\nx1=x1+(xc-xw/2);\nx2=x1+xw-1;\ny1=y1+(yc-yw/2);\ny2=y1+yw-1;\nif (x1 < 0)\n{ x1 = 0;\n   x2 = x1+xw-1; }\nif (x2 >= wi)\n{ x2 = wi-1;\n   x1 = x2-xw+1; }\nif (y1 < 0)\n{ y1 = 0;\n   y2 = y1+yw-1; }\nif (y2 >= ht)\n{ y2 = ht -1;\n   y1 = y2-yw+1; }"("i"=w581, "xc"=w573, "yc"=w574, "wi"=w570, "ht"=w569) -> ("x1"=w580:dbl, "y1"=w579:dbl, "x2"=w578:dbl, "y2"=w577:dbl, "xw"=w572:dbl, "yw"=w571:dbl)
                      n136 = Build Array(w580, w579, w578, w577) -> (w576:dbl[])
                      n137 = To Unsigned Word Integer(number=w576) -> (unsigned 16bit integer=w575:u16[])
                    }
                  }
                  n138 = Add(x=w528, y=w518) -> (x+y=w520:dbl)
                  n139 = Add(x=w517, y=w529) -> (x+y=w519:dbl)
                  n140 = case shown="True" w514 {
                    tunnel: w527 -> [w533 w539]
                    tunnel: [w532 w538] -> w526
                    tunnel: [w533 w537] -> w525
                    tunnel: w524 -> [w532 w536]
                    tunnel: w520 -> [_ w535]
                    tunnel: w519 -> [_ w534]
                    frame False {
                    }
                    frame True {
                      n141 = To Long Integer(number=w534) -> (32bit integer=w542:i32)
                      n142 = To Long Integer(number=w535) -> (32bit integer=w541:i32)
                      n143 = for {
                        N: 5 -> [_]
                        tunnel: w542 -> [w552]
                        tunnel: w541 -> [w551]
                        tunnel: w539 -> [w546]
                        shift-right: [w544] -> w538
                        shift-left: w536 -> [w545]
                        tunnel: [w543] -> w537
                        i -> [w553]
                        n144 = case shown="4" w553 {
                          tunnel: w552 -> [w555 w556 w560 w562 w566]
                          tunnel: [w555 w556 w561 w562 w567] -> w550
                          tunnel: w551 -> [w554 w558 w559 w563 w565]
                          tunnel: [w554 w557 w559 w564 w565] -> w549
                          frame 0, Default {
                          }
                          frame 1 {
                            n145 = Increment(x=w558) -> (x+1=w557:i32)
                          }
                          frame 2 {
                            n146 = Increment(x=w560) -> (x+1=w561:i32)
                          }
                          frame 3 {
                            n147 = Decrement(x=w563) -> (x-1=w564:i32)
                          }
                          frame 4 {
                            n148 = Decrement(x=w566) -> (x-1=w567:i32)
                          }
                        }
                        n149 = Bundle(w549, w550) -> (w547:cluster{i32, i32})  [unwired: 1 out]
                        n150 = call "IMAQ Overlay Points"("Color"=u32 16711680, "error in (no error)"=w545, "Point"=w547, "Image"=w546) -> ("error out"=w544:errorcluster, "Image Out"=w543:T9)  [unwired: 2 in, 4 out]
                      }
                    }
                  }
                }
              }
            }
            frame #5 {
              # "write line to output file"
              n151 = Or(x=w582, y="Write record when no fit?") -> (x .or. y?=w584:bool)
              n152 = case shown="True" w584 {
                tunnel: w594 -> [_ w609]
                tunnel: w593 -> [_ w607]
                tunnel: w592 -> [_ w613]
                tunnel: w591 -> [_ w599]
                tunnel: w590 -> [_ w618]
                tunnel: w589 -> [_ w615]
                tunnel: w588 -> [_ w603]
                tunnel: w587 -> [_ w601]
                tunnel: w586 -> [_ w611]
                tunnel: w585 -> [_ w612]
                tunnel: w582 -> [_ w597]
                frame False {
                }
                frame True {
                  # "delete CR"
                  n153 = for {
                    tunnel: w613 -> [w642] mode=indexing
                    tunnel: [w641] -> w605 mode=indexing
                    tunnel: [ext 0.0 ("Start frame")] -> w596 mode=indexing
                    n154 = Unbundle By Name(w642) -> ("Initial Val."=w641:dbl)
                  }
                  n155 = case shown="False" w597 {
                    tunnel: [w629 w639] -> w610
                    tunnel: w611 -> [w629 w639]
                    tunnel: [w628 w638] -> w608
                    tunnel: w609 -> [w628 w638]
                    tunnel: [w627 w637] -> w606
                    tunnel: w607 -> [w627 w637]
                    tunnel: [w631 w636] -> w604
                    tunnel: w605 -> [_ w636]
                    tunnel: [w632 w635] -> w602
                    tunnel: w603 -> [_ w635]
                    tunnel: [w632 w634] -> w600
                    tunnel: w601 -> [_ w634]
                    tunnel: [-1.0 ("mse") w633] -> w598
                    tunnel: w599 -> [_ w633]
                    tunnel: w596 -> [w631 _]
                    frame False {
                      w632 = u32 0 ("Start frame")
                    }
                    frame True {
                    }
                  }
                  n156 = Increment(x=w608) -> (x+1=w625:i32)
                  n157 = Build Array(w610, w625, w606) -> (w624:u32[])
                  n158 = Build Array (concatenate)(w604, w602, w600, w598, w612) -> (w623:ext[])
                  n159 = Array To Spreadsheet String(delimiter (Tab)=w615, array=w624, 3:"%d" ("format string")) -> (spreadsheet string=w617:string)
                  n160 = Array To Spreadsheet String(delimiter (Tab)=w615, array=w623, 3:"%f" ("format string")) -> (spreadsheet string=w621:string)
                  n161 = Search and Replace String(input string=w617, search string="\r\n", replace string=w615) -> (result string=w616:string)  [unwired: 1 in, 7 out]
                  n162 = Concatenate Strings(w616, w621) -> (w620:string)
                  n163 = Write to Binary File(file (use dialog)=w618, data=w620, 5:FALSE ("prepend array or string size? (T)")) -> (error out=w619:errorcluster)  [unwired: 1 in, 4 out]
                  n164 = call <vilib>:"Simple Error Handler.vi"("error in (no error)"=w619) -> ()  [unwired: 1 in, 8 out]
                }
              }
            }
            frame #6 {
              n165 = local read "Move AOIs?"() -> (w648:bool)
              n166 = for {
                tunnel: w644 -> [w652] mode=indexing
                tunnel: [w651] -> w643 mode=indexing
                n167 = Unbundle By Name(w652) -> ("Initial Val."=w651:dbl)
              }
              "Fit" <- w643
              n168 = And(x=w650, y=w648) -> (x .and. y?=w649:bool)
              n169 = case shown="True" w649 {
                tunnel: w644 -> [w653 w657]
                tunnel: [w653 w656] -> w647
                tunnel: w646 -> [_ w655]
                tunnel: w645 -> [_ w654]
                frame False {
                }
                frame True {
                  # "update xc and yc parameters (to aoi center) to compensate for aoi movement."
                  n170 = for {
                    tunnel: w657 -> [w664] mode=indexing
                    tunnel: [w660] -> w656 mode=indexing
                    tunnel: w655 -> [w659]
                    tunnel: w654 -> [w658]
                    n171 = Unbundle By Name(w664) -> ("Name"=w665:string, "Initial Val."=w662:dbl)
                    n172 = case shown="Default" w665 {
                      selector: w665 -> [w667 w671 w675]
                      tunnel: [w667 w671 w675] -> w663
                      tunnel: w662 -> [w666 _ _]
                      tunnel: [w666 w670 w674] -> w661
                      tunnel: w659 -> [_ w668 _]
                      tunnel: w658 -> [_ _ w672]
                      frame Default {
                      }
                      frame "xc" {
                        n173 = Divide(x=w668, y=2.0) -> (x/y=w670:dbl)
                      }
                      frame "yc" {
                        n174 = Divide(x=w672, y=2.0) -> (x/y=w674:dbl)
                      }
                    }
                    n175 = Bundle By Name(cluster=w664, "Name"=w663, "Initial Val."=w661) -> (w660:T14)
                  }
                }
              }
            }
          }
          n176 = Or(x=w309, y=w308) -> (x .or. y?=w310:bool)
        }
        "MSEs" <- w261
        n177 = Increment(x=w240) -> (x+1=w272:u32)
        n178 = case shown="True" w234 {
          tunnel: w258 -> [w274 w295]
          tunnel: w251 -> [w273 w294]
          tunnel: [w274 w281] -> w236
          tunnel: w248 -> [_ w291]
          tunnel: w247 -> [_ w290]
          tunnel: [w273 w280] -> w235
          tunnel: "White level" -> [_ w279]
          tunnel: "Black level" -> [_ w278]
          tunnel: w229 -> [_ w277]
          tunnel: w225 -> [_ w275]
          frame False {
          }
          frame True {
            w288 = 13 ("Window Number (0...15)")
            w286 = 1 items=["Hide", "Show", "No change"] ("Scrollbars (No change)")
            # "display tracking results graphical window"
            n179 = call "IMAQ Copy Overlay"("error in (no error)"=w295, "Image Dst"=w294, "Image Src"=w290) -> ("error out"=w293:errorcluster, "Image Dst Out"=w292:T9)  [unwired: 1 in, 6 out]
            n180 = call "IMAQ Copy Overlay"("error in (no error)"=w293, "Image Dst"=w292, "Image Src"=w291) -> ("error out"=w282:errorcluster, "Image Dst Out"=w284:T9)  [unwired: 1 in, 6 out]
            n181 = Equal To 0?(x=w275) -> (x = 0?=w276:bool)
            n182 = call "Glimpse display gain-offset old.vi"("White level"=w279, "Black level"=w278, "Pixel depth"=w277, "Window Number (0...15)"=w288, "error in"=w282, "Resize to Image Size? (Y)"=w276, "Window Title"="Tracking Results" ("Title"), "Image In"=w284) -> ("error out"=w289:errorcluster, "Image Out"=w280:T9)  [unwired: 2 out]
            n183 = call "IMAQ WindMove"("Window Number (0...15)"=w288, "Coordinates (screen)"=cluster{"X Position":i32, "Y Position":i32} {"X Position"=90, "Y Position"=0}, "error in (no error)"=w289) -> ("error out"=w285:errorcluster)  [unwired: 1 in, 2 out]
            n184 = call "IMAQ WindSetup"("Scrollbars (No change)"=w286, "Window Number (0...15)"=w288, "error in (no error)"=w285) -> ("error out"=w281:errorcluster)  [unwired: 4 in, 4 out]
          }
        }
        "Frame Number" <- w240
      }
      n185 = call "IMAQ Create"("Image Name"="fctemp2", "Image Type"=w162, "error in (no error)"=w167) -> ("New Image"=w163:T9, "error out"=w166:errorcluster)  [unwired: 1 in, 1 out]
      n186 = call "Make 16 to 8 LUT.vi"("Black level"=w168, "White level"=w169) -> ("Lookup Table"=w170:i16[])
      n187 = call "IMAQ UserLookup"("Image Src"=w165, "Lookup Table"=w170, "error in (no error)"=w166) -> ("Image Dst Out"=w164:T9, "error out"=w161:errorcluster)  [unwired: 2 in, 2 out]
      n188 = call "Change file name extension.vi"("New Extension (no period)"="jpg", "Path String In"=w151) -> ("New Path Out"=w150:path)  [unwired: 3 out]
      n189 = call "IMAQ Cast Image"("Image Type"=w162, "error in (no error)"=w161, "Image Dst"=w163, "Image Src"=w164) -> ("error out"=w160:errorcluster, "Image Dst Out"=w155:T9)  [unwired: 2 in, 4 out]
      n190 = call "IMAQ Create"("Image Name"="fctemp", "Image Type"=w174, "error in (no error)"=w160) -> ("New Image"=w157:T9, "error out"=w173:errorcluster)  [unwired: 1 in, 1 out]
      n191 = call "IMAQ Merge Overlay"("error in (no error)"=w173, "Image Dst"=w157, "Image Src"=w155) -> ("error out"=w159:errorcluster, "Image Dst Out"=w156:T9)  [unwired: 2 in, 5 out]
      n192 = Strip Path(path=w150) -> (name=w136:string)  [unwired: 1 out]
      n193 = Concatenate Strings("" ("string"), w136) -> (w134:string)
      n194 = stacked-sequence {
        tunnel: w178 -> [_]
        tunnel: w177 -> [w224]
        tunnel: w151 -> [w218]
        tunnel: w176 -> [w214]
        tunnel: [w218] -> _
        tunnel: w134 -> [w195]
        frame #0 {
          n195 = Close File(refnum=w224) -> ()  [unwired: 1 in, 2 out]
          n196 = Get Date/Time In Seconds() -> (seconds since 1Jan1904=w196:timestamp)
          n197 = call-poly <vilib>:"Append Report Text.vi"("report in"=w214, "text"="Fitting ended ", "append on new line? (F)"=TRUE) -> ("report out"=w197:T10, "error out"=w198:errorcluster)  [unwired: 3 in, 8 out]
          n198 = To Double Precision Float(number=w196) -> (double precision float=w217:dbl)
          n199 = Format Date/Time String(time format string (%c)="%Y%m%d_%H%M%S", seconds (now)=w217) -> (date/time string=w211:string)  [unwired: 1 out]
          n200 = call-poly <vilib>:"Append Report Text.vi"("report in"=w197, "text"=w211, "append on new line? (F)"=FALSE, "error in (no error)"=w198) -> ("report out"=w199:T10, "error out"=w200:errorcluster)  [unwired: 2 in, 8 out]
          n201 = call-dynamic "New Report Line.vi"("report in"=w199, "error in (no error)"=w200) -> ("report out"=w212:T10, "error out"=w201:errorcluster)  [unwired: 1 in, 11 out]
          n202 = call-dynamic "Append Horizontal Line to Report.vi"("report in"=w212, "align (default)"=HTML_Report_Text_Alignment."CENTER", "error in (no error)"=w201) -> ("report out"=w202:T10, "error out"=w205:errorcluster)  [unwired: 5 in, 6 out]
          n203 = call-dynamic "New Report Line.vi"("report in"=w202, "error in (no error)"=w205) -> ("report out"=w203:T10, "error out"=w206:errorcluster)  [unwired: 1 in, 11 out]
          n204 = call-poly <vilib>:"Append Image to Report.vi"("report in"=w203, "alignment (default)"=HTML_Report_Image_Alignment."LEFT", "path or URL of image"=w195, "error in (no error)"=w206) -> ("report out"=w204:T10, "error out"=w207:errorcluster)  [unwired: 2 in, 8 out]
          n205 = call "Change file name extension.vi"("New Extension (no period)"="html", "Path String In"=w218) -> ("New Path Out"=w223:path)  [unwired: 3 out]
          n206 = call-dynamic "Save Report to File.vi"("report in"=w204, "report file path"=w223, "error in (no error)"=w207) -> ("report out"=w221:T10, "error out"=w222:errorcluster)  [unwired: 2 in, 9 out]
          n207 = call-dynamic "Dispose Report.vi"("report in"=w221, "error in (no error)"=w222) -> ("error out"=w220:errorcluster)  [unwired: 3 in, 10 out]
          n208 = call <vilib>:"Simple Error Handler.vi"("error in (no error)"=w220) -> ()  [unwired: 1 in, 8 out]
        }
      }
      n209 = call "IMAQ Write JPEG File"("error in (no error)"=w159, "File Path"=w150, "Image"=w156) -> ("error out"=w158:errorcluster)  [unwired: 2 in, 3 out]
      n210 = call "IMAQ Dispose"("Image"=w156, "error in (no error)"=w158) -> ("error out"=w154:errorcluster)  [unwired: 1 in, 3 out]
      n211 = call "IMAQ Dispose"("Image"=w155, "error in (no error)"=w154) -> ("error out"=w153:errorcluster)  [unwired: 1 in, 3 out]
      n212 = call "IMAQ Dispose"("Image"=w165, "error in (no error)"=w153) -> ("error out"=w183:errorcluster)  [unwired: 1 in, 3 out]
      n213 = call "IMAQ Dispose"("Image"=w185, "error in (no error)"=w183) -> ("error out"=w181:errorcluster)  [unwired: 1 in, 3 out]
      n214 = call "IMAQ Dispose"("Image"=w180, "error in (no error)"=w181) -> ("error out"=w142:errorcluster)  [unwired: 1 in, 3 out]
      n215 = Open VI Reference(vi path=path "Fit one AOI.vi", error in (no error)=w142) -> (vi reference=w148:refnum<vi>, error out=w147:errorcluster)  [unwired: 4 out]
      n216 = property class="VI"(reference=w148, error in=w147, "Front Panel Window:Open"=FALSE) -> (reference out=w146:refnum<vi>, error out=w145:errorcluster)
      n217 = Close Reference(reference=w146, error in (no error)=w145) -> (error out=w141:errorcluster)
      n218 = call "Glimpse error handler.vi"("error in"=w141, "Dialog box?"=TRUE) -> ()  [unwired: 6 out]
    }
  }
